vi "Newton_New dx.vi"(9 "dx in":dbl, 10 "P'(x0)":dbl, 11 "P(x0)":dbl) -> (3 "dx out":dbl)   [LabVIEW 2014, in "NI_AALPro.lvlib"]
uses:
  NI_AALPro.lvlib
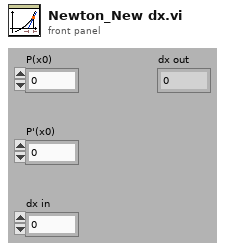
[diagram p1: front panel]
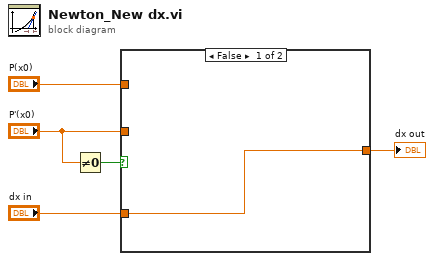
[diagram p0: block diagram]
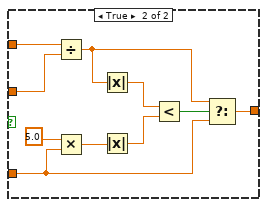
[diagram p2: hidden frame]
diagram:
  n1 = Not Equal To 0?(x="P'(x0)") -> (x != 0?=w3:bool)
  n2 = case shown="False" w3 {
    tunnel: "P'(x0)" -> [_ w15]
    tunnel: "P(x0)" -> [_ w16]
    tunnel: "dx in" -> [w6 w8]
    tunnel: [w6 w9] -> w1
    frame False {
    }
    frame True {
      n3 = Divide(x=w16, y=w15) -> (x/y=w10:dbl)
      n4 = Multiply(x=5.0 ("y"), y=w8) -> (x*y=w13:dbl)
      n5 = Absolute Value(x=w10) -> (abs(x)=w14:dbl)
      n6 = Absolute Value(x=w13) -> (abs(x)=w12:dbl)
      n7 = Less?(x=w14, y=w12) -> (x < y?=w11:bool)
      n8 = Select(t=w10, s=w11, f=w8) -> (s? t:f=w9:dbl)
    }
  }
  "dx out" <- w1
